vi "PID_2Chan_V4_Ramps.vi"() -> ()   [LabVIEW 2016]
uses:
  <vilib>/addons/control/pid/pid.llb/PID Advanced (DBL Array).vi
  <vilib>/addons/control/pid/pid.llb/PID Parameter Manager (DBL Array).vi
  <vilib>/addons/control/pid/pid.llb/PID Derivative Action Buffered (DBL Array).vi
  <vilib>/addons/control/pid/pid.llb/PID Get Advanced Error (DBL Array).vi
  <vilib>/addons/control/pid/pid.llb/PID Integral Action Buffered (DBL Array).vi
  <vilib>/addons/control/pid/pid.llb/PID Resize 1D Array.vi
  <vilib>/addons/control/pid/pid.llb/PID Get Advanced Error (DBL).vi
  <userlib>/Fluigent/Fluigent MFCS/FluigentMFCS_Full.llb/MFCS_EZ Detect.vi
  <userlib>/Fluigent/Fluigent MFCS/FluigentMFCS_Full.llb/MFCS_EZ Initialization.vi
  <userlib>/Fluigent/Fluigent MFCS/FluigentMFCS_Full.llb/MFCS_EZ Read All Channels Pressure.vi
  <userlib>/Fluigent/Fluigent MFCS/FluigentMFCS_Full.llb/MFCS_EZ Write Channel Pressure.vi
  <userlib>/Fluigent/Fluigent MFCS/FluigentMFCS_Full.llb/MFCS_EZ Close.vi
  <vilib>/addons/control/pid/NI_PID_pid.lvlib
  <vilib>/Analysis/NI_AALBase.lvlib
  <vilib>/Analysis/baseanly.llb/Mean (DBL).vi
panel:
  in  "setpoint profile":cluster{"time (s)":dbl, "setpoint":dbl}[](array[cluster]) {"setpoint" format="%.2f"; "time (s)" format="%.3f"}
  in  "Ramp?":bool
  in  "output cluster":T1
  out "Set Pressure":dbl[](array[numeric])=[400.0, 400.0]
  in  "linearity":dbl[](array[numeric])=[0.10000000000000003, 0.6000000000000001] format="%.2f"
  out "Flow 1 plot 2":cluster{"[0]":dbl, "[1]":dbl}(graph)={"[0]"=400.0, "[1]"=636.4874575000703}
  out "Flow Rates":dbl[](array[numeric])=[1099.9989421021717, 636.4874575000703]
  in  "FTot PID gains":cluster{"P":dbl, "I":dbl, "D":dbl}={"P"=0.01, "I"=0.0, "D"=0.0} {"D" format="%.6f"; "I" format="%.3f"; "P" format="%.5f"}
  in  "Ftot Setpoint":dbl=400.0
  in  "Vals to display":dbl=1235.0
  out "Flow 1 plot":cluster{"[0]":dbl, "[1]":dbl}(graph)={"[0]"=1099.9989421021717, "[1]"=300.0}
  out "Ferr":T2(graph)={"output[0]"=-2.2986299232843663, "output[1]"=-0.9866301071552578, "output[2]"=0.0}
  out "Pressures":dbl[](array[numeric])=[404.58697509765625, 396.3816223144531]
  in  "F1 PID gains":cluster{"P":dbl, "I":dbl, "D":dbl}={"P"=0.001, "I"=0.0, "D"=0.001} {"D" format="%.6f"; "I" format="%.3f"; "P" format="%.5f"}
  in  "reset Averging":bool
  in  "Set current Pressure\n to manual pressure":bool
  out "Pressures":T3(graph)={"[0]"=404.58697509765625, "[1]"=396.3816223144531, "[2]"=400.0, "[3]"=400.0}
  in  "stop":bool=TRUE
  in  "Control Valves":enum16{"1", "2", "3", "4", "5", "6", "7", "8"}[](array[ring])=[enum."7", enum."8"]
  in  "Pressure Channels":i16[](array[numeric])=[2, 3]
  in  "Manual Pressure Set":dbl[](array[numeric])=[400.0, 400.0] format="%_7g"
  in  "PID On":bool
  in  "reinitialize? (F)":bool
  in  "F1 Setpoint":dbl=300.0
  in  "Add Ctrl?":bool
  in  "Boards":enum16{"A", "B", "C"}[](array[ring])=[enum."A", enum."A"]
  in  "Valves":enum16{"1", "2", "3", "4", "5", "6", "7", "8"}[](array[ring])=[enum."5", enum."1"]
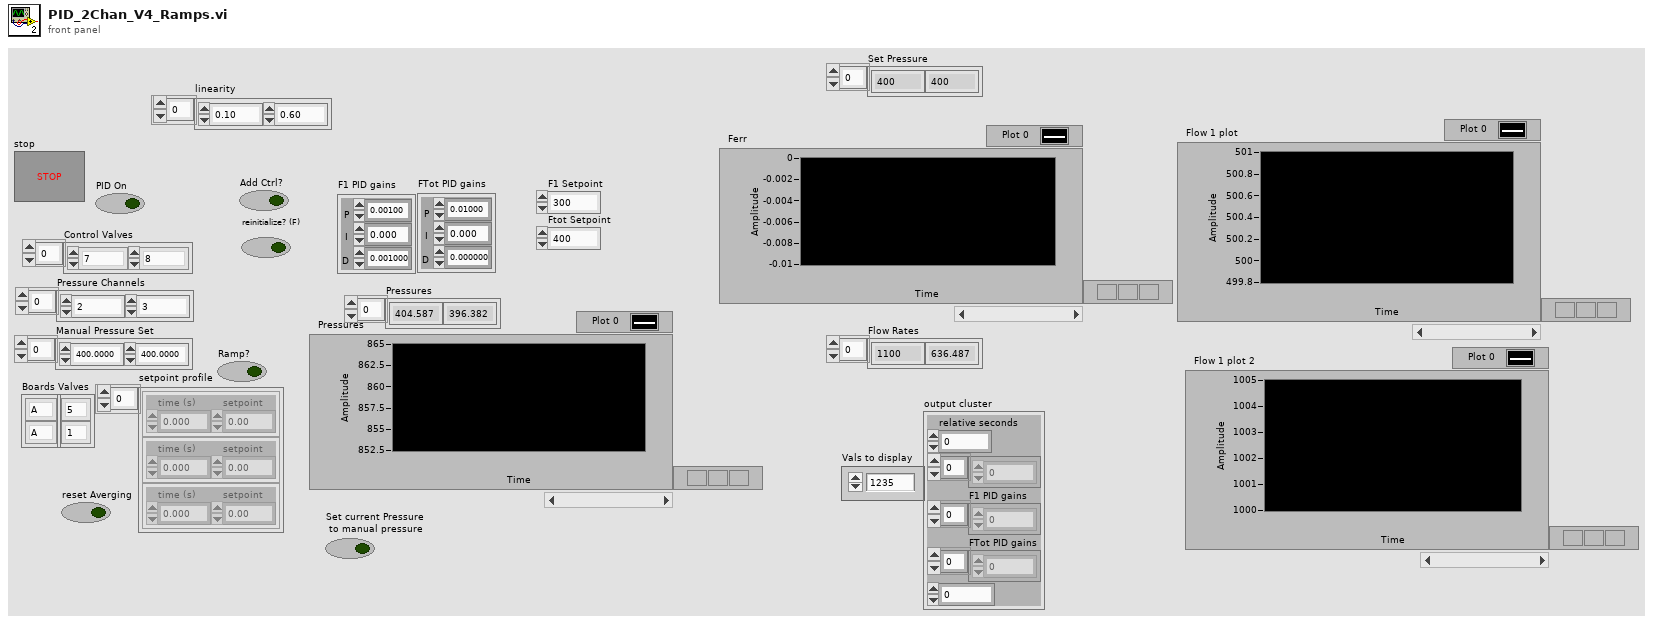
[diagram p1: front panel]
types:
  T1 = cluster{"relative seconds":dbl, "Pressures":dbl[], "F1 PID gains":dbl[], "FTot PID gains":dbl[], "PID On?":i16}
  T2 = cluster{"output[0]":dbl, "output[1]":dbl, "output[2]":dbl}
  T3 = cluster{"[0]":dbl, "[1]":dbl, "[2]":dbl, "[3]":dbl}
  T4 = cluster{"setpoint high":dbl, "setpoint low":dbl}[]
  T5 = typedef "_EZmfcsSN.ctl" = u16
  T6 = typedef "_EZmfcsRefNum.ctl" = refnum<k1>
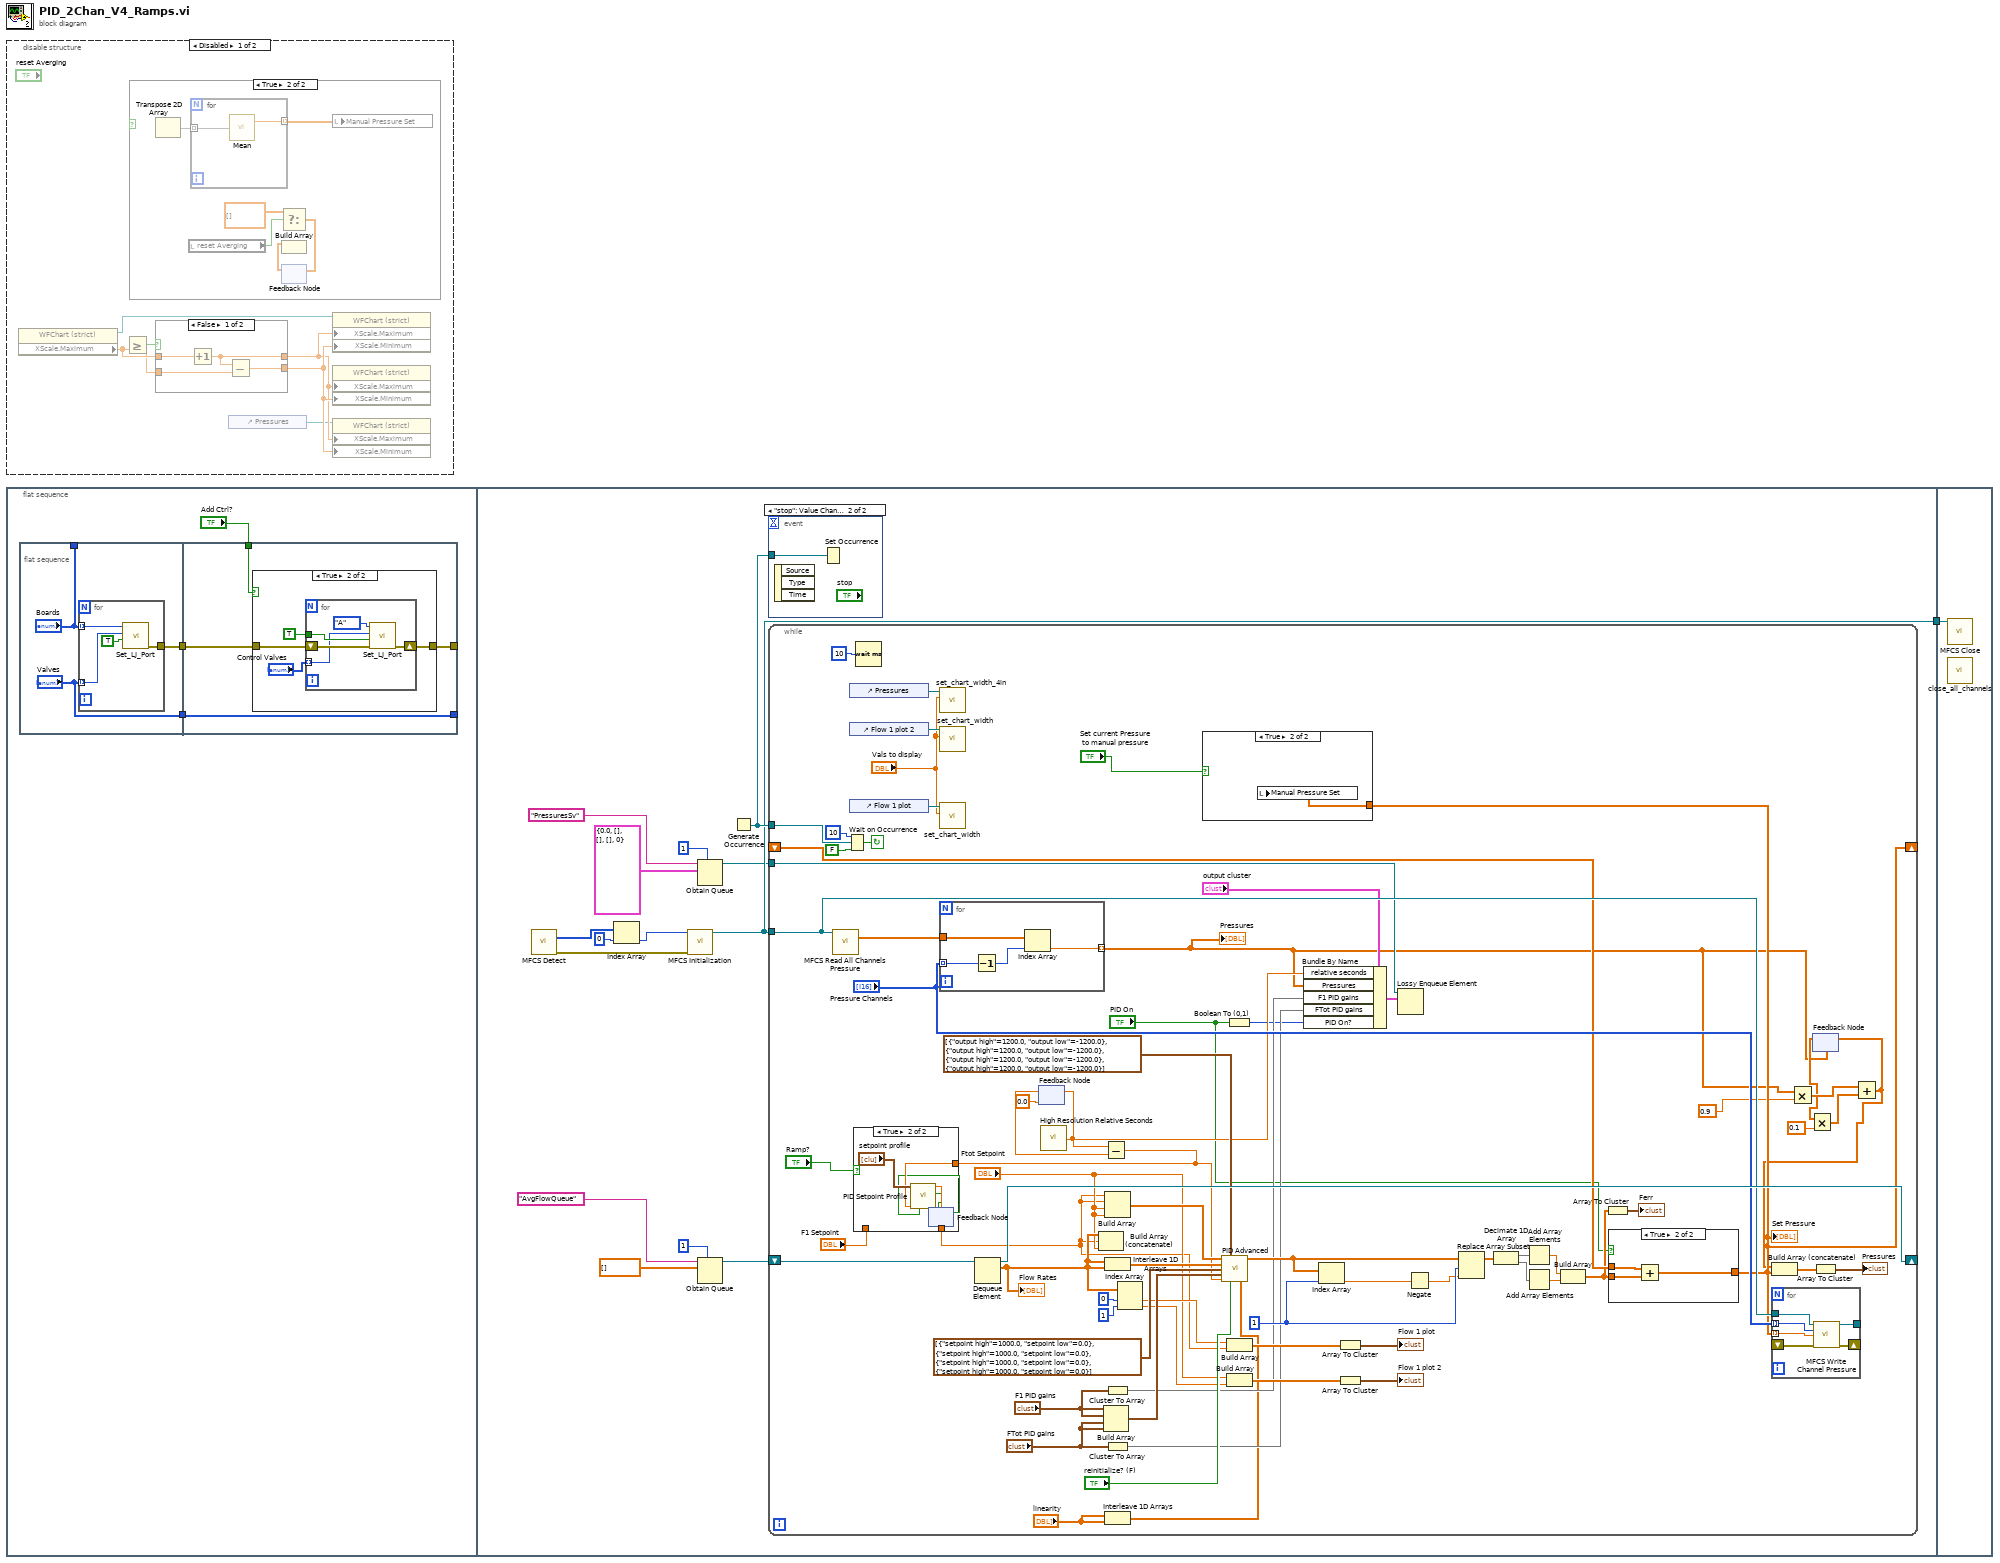
[diagram p0: block diagram]
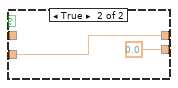
[diagram p2: hidden frame]
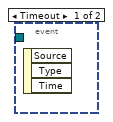
[diagram p6: hidden frame]
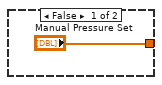
[diagram p9: hidden frame]
diagram:
  n1 = disable-structure shown="Disabled" {
    frame Disabled {
      n2 = property on="Property Node" class="WFChart (strict)"() -> (reference=w5:refnum<vi>, reference out=w6:refnum<vi>, "XScale.Maximum"=w4:dbl)  [unwired: 1 in, 1 out]
      n3 = Greater Or Equal?(y=w4) -> (x=w2:dbl, x >= y?=w3:bool)
      n4 = case shown="True" w11 {
        frame False {
        }
        frame True {
          n5 = Transpose 2D Array() -> (transposed array=w21:dbl[][])  [unwired: 1 in]
          n6 = local read "reset Averging"() -> (w22:bool)
          n7 = for {
            tunnel: w21 -> [w25] mode=indexing
            tunnel: [w24] -> w18 mode=indexing
            n8 = call-poly <vilib>:"Mean.vi"("X"=w25) -> ("mean"=w24:dbl)  [unwired: 1 out]
          }
          n9 = Select(t=dbl[][] [] ("appended array"), s=w22) -> (s? t:f=w19:dbl[][])  [unwired: 1 in]
          n10 = feedback-in #1(w19) -> ()
          n11 = feedback #1() -> (w23:dbl[][])  [unwired: 1 in]
          n12 = Build Array(w23) -> ()  [unwired: 1 in, 1 out]
          n13 = local write "Manual Pressure Set"(w18) -> ()
        }
      }
      n14 = case shown="False" w3 {
        tunnel: w2 -> [w13 w17]
        tunnel: w4 -> [w15 _]
        tunnel: [w12 w17] -> w9
        tunnel: [w14 0.0] -> w10
        frame False {
          n15 = Increment(x=w15) -> (x+1=w12:dbl)
          n16 = Subtract(x=w12, y=w13) -> (x-y=w14:dbl)
        }
        frame True {
        }
      }
      n17 = control-ref of="Pressures"() -> (w7:refnum<vi>)
      n18 = property on="Property Node" class="WFChart (strict)"(reference=w6, "XScale.Maximum"=w9, "XScale.Minimum"=w10) -> ()  [unwired: 1 in, 2 out]
      n19 = property on="Property Node" class="WFChart (strict)"("XScale.Maximum"=w9, "XScale.Minimum"=w10) -> (reference=w8:refnum<vi>)  [unwired: 1 in, 2 out]
      n20 = property on="Property Node" class="WFChart (strict)"(reference=w7, "XScale.Maximum"=w9, "XScale.Minimum"=w10) -> ()  [unwired: 1 in, 2 out]
    }
    frame Enabled {
    }
  }
  n21 = flat-sequence {
    tunnel: [w54] -> w1
    tunnel: w1 -> [w157]
    frame #0 {
      n22 = flat-sequence {
        tunnel: ["Boards"] -> _
        tunnel: [w31] -> w28
        tunnel: ["Valves"] -> w27
        tunnel: [w39] -> _
        tunnel: [w37] -> _
        tunnel: w28 -> [w38]
        tunnel: w27 -> [w39]
        tunnel: "Add Ctrl?" -> [w36]
        frame #0 {
          n23 = for {
            tunnel: "Valves" -> [w35] mode=indexing
            tunnel: "Boards" -> [w34] mode=indexing
            tunnel: [w32] -> w31
            n24 = call "Set_LJ_Port.vi"("State"=TRUE, "Channel"=w35, "Flowboard"=w34) -> ("error out"=w32:errorcluster)  [unwired: 8 in]
          }
        }
        frame #1 {
          n25 = case shown="True" w36 {
            tunnel: w38 -> [w40 w44]
            tunnel: [w40 w43] -> w37
            frame False {
            }
            frame True {
              n26 = for {
                tunnel: TRUE ("State") -> [w47]
                shift-right: [w48] -> w43
                shift-left: w44 -> [w49]
                tunnel: "Control Valves" -> [w46] mode=indexing
                n27 = call "Set_LJ_Port.vi"("error in"=w49, "State"=w47, "Channel"=w46, "Flowboard"=enum16{"A", "B", "C"}."A") -> ("error out"=w48:errorcluster)  [unwired: 7 in]
              }
            }
          }
        }
      }
    }
    frame #1 {
      n28 = call-poly <userlib>:"MFCS Detect.vi"() -> ("[SN MFCS_EZ]"=w63:T5[], "error out"=w61:errorcluster)  [unwired: 14 in]
      n29 = Index Array(array=w63, index=0) -> (element=w62:T5)
      n30 = call-poly <userlib>:"MFCS Initialization.vi"("SN MFCS_EZ"=w62, "error in (no error)"=w61) -> ("MFCS_EZ"=w54:T6)  [unwired: 11 in, 2 out]
      n31 = Obtain Queue(max queue size (-1, unlimited)=1, name (unnamed)="PressuresSv", element data type=T1 {"relative seconds"=0.0, "Pressures"=[], "F1 PID gains"=[], "FTot PID gains"=[], "PID On?"=0} ("output cluster")) -> (queue out=w52:refnum<queue>)  [unwired: 2 in, 2 out]
      n32 = Obtain Queue(max queue size (-1, unlimited)=1, name (unnamed)="AvgFlowQueue", element data type=dbl[] [] ("appended array")) -> (queue out=w57:refnum<queue>)  [unwired: 2 in, 2 out]
      n33 = Generate Occurrence() -> (w56:refnum<k4>)
      n34 = event shown="[1] \"stop\": Value Change" {
        selector: _ -> [_ _]
        dyn-events: _ -> [_ _]
        timeout: _ -> [_ _]
        tunnel: w56 -> [_ w64]
        event Timeout {
          n35 = event-data() -> ()  [unwired: 1 in, 3 out]
        }
        event "stop": Value Change {
          n36 = event-data() -> ()  [unwired: 1 in, 3 out]
          n37 = Set Occurrence(w64) -> ()
        }
      }
      n38 = while {
        shift-right: [w134] -> _
        shift-left: w57 -> [w135]
        tunnel: w56 -> [w121]
        tunnel: w54 -> [w110]
        shift-right: [w73] -> _
        shift-left: _ -> [w105]
        tunnel: w52 -> [w96]
        stop <- w120 continue-if-true
        w128 = 1 ("index")
        n39 = call-poly <userlib>:"MFCS Read All Channels Pressure.vi"("MFCS_EZ"=w110) -> ("All Channels Pressure"=w108:dbl[])  [unwired: 12 in, 2 out]
        n40 = Wait on Occurrence(1:FALSE ("ignore previous (T)"), 2:w121, 3:10 ("ms timeout (-1)")) -> (0:w120:bool)
        n41 = control-ref of="Pressures"() -> (w107:refnum<vi>)
        n42 = control-ref of="Flow 1 plot 2"() -> (w90:refnum<vi>)
        n43 = control-ref of="Flow 1 plot"() -> (w89:refnum<vi>)
        n44 = Wait (ms)(milliseconds to wait=u32 10) -> ()  [unwired: 1 out]
        n45 = call "set_chart_width_4in.vi"("Values to Display"="Vals to display", "Ref In"=w107) -> ()  [unwired: 10 in]
        n46 = call "set_chart_width.vi"("Values to Display"="Vals to display", "Ref In"=w90) -> ()  [unwired: 10 in]
        n47 = call "set_chart_width.vi"("Values to Display"="Vals to display", "Ref In"=w89) -> ()  [unwired: 10 in]
        n48 = for {
          tunnel: "Pressure Channels" -> [w145] mode=indexing
          tunnel: w108 -> [w146]
          tunnel: [w143] -> w65 mode=indexing
          n49 = Decrement(x=w145) -> (x-1=w144:i16)
          n50 = Index Array(array=w146, index=w144) -> (element=w143:dbl)
        }
        "Pressures" <- w65
        n51 = Dequeue Element(queue=w135) -> (queue out=w134:refnum<queue>, element=w101:dbl[])  [unwired: 2 in, 2 out]
        "Flow Rates" <- w101
        n52 = feedback #2(0.0 ("relative seconds")) -> (w130:dbl)
        n53 = call <vilib>:"High Resolution Relative Seconds.vi"() -> ("relative seconds"=w95:dbl)
        n54 = feedback-in #2(w95) -> ()
        n55 = Subtract(x=w95, y=w130) -> (x-y=w77:dbl)
        n56 = case shown="True" "Ramp?" {
          tunnel: w77 -> [_ w141]
          tunnel: [w137 w140] -> w76
          tunnel: "F1 Setpoint" -> [w137 _]
          frame False {
          }
          frame True {
            n57 = feedback #3() -> (w138:bool)  [unwired: 1 in]
            n58 = call <vilib>:"PID Setpoint Profile.vi"("reinitialize? (F)"=w138, "dt (s)"=w141, "setpoint profile"="setpoint profile") -> ("profile complete?"=w139:bool, "setpoint"=w140:dbl)  [unwired: 3 in, 2 out]
            n59 = feedback-in #3(w139) -> ()
          }
        }
        n60 = Build Array (concatenate)(w101, w76, "Ftot Setpoint") -> ()  [unwired: 1 out]
        n61 = Build Array("F1 PID gains", "F1 PID gains", "FTot PID gains", "FTot PID gains") -> (w124:cluster{"P":dbl, "I":dbl, "D":dbl}[])
        n62 = Build Array(w76, w76, "Ftot Setpoint", "Ftot Setpoint") -> (w118:dbl[])
        n63 = Interleave 1D Arrays(w101, w101) -> (w112:dbl[])
        n64 = Cluster To Array(cluster="F1 PID gains") -> (array=w94:dbl[])
        n65 = Cluster To Array(cluster="FTot PID gains") -> (array=w93:dbl[])
        n66 = Interleave 1D Arrays("linearity", "linearity") -> (w81:dbl[])
        n67 = Index Array(array=w101, index #1=0 ("index"), index #2=1 ("index")) -> (element #1=w87:dbl, element #2=w85:dbl)
        n68 = call-poly <vilib>:"PID Advanced.vi"("setpoint"=w118, "output range"=cluster{"output high":dbl, "output low":dbl}[] [{"output high"=1200.0, "output low"=-1200.0}, {"output high"=1200.0, "output low"=-1200.0}, {"output high"=1200.0, "output low"=-1200.0}, {"output high"=1200.0, "output low"=-1200.0}], "process variable"=w112, "setpoint range"=T4 [{"setpoint high"=1000.0, "setpoint low"=0.0}, {"setpoint high"=1000.0, "setpoint low"=0.0}, {"setpoint high"=1000.0, "setpoint low"=0.0}, {"setpoint high"=1000.0, "setpoint low"=0.0}], "PID gains"=w124, "dt (s)"=w77, "reinitialize? (F)"="reinitialize? (F)", "linearity"=w81) -> ("output"=w125:dbl[])  [unwired: 6 in, 1 out]
        n69 = Boolean To (0,1)(Boolean="PID On") -> (0, 1=w91:i16)
        n70 = Build Array(w87, w76) -> (w100:dbl[])
        n71 = Build Array("Ftot Setpoint", w85) -> (w98:dbl[])
        n72 = Bundle By Name(cluster="output cluster", "relative seconds"=w95, "Pressures"=w65, "F1 PID gains"=w94, "FTot PID gains"=w93, "PID On?"=w91) -> (w79:T1)
        n73 = Index Array(array=w125, index=w128) -> (element=w127:dbl)
        n74 = Array To Cluster(array=w100) -> (cluster=→"Flow 1 plot":cluster{"[0]":dbl, "[1]":dbl})
        n75 = Array To Cluster(array=w98) -> (cluster=→"Flow 1 plot 2":cluster{"[0]":dbl, "[1]":dbl})
        n76 = Lossy Enqueue Element(queue=w96, element=w79) -> ()  [unwired: 1 in, 4 out]
        n77 = Negate(x=w127) -> (-x=w126:dbl)
        n78 = Replace Array Subset(array=w125, new element=w126, index=w128) -> (w117:dbl[])
        n79 = Decimate 1D Array(w117) -> (w116:dbl[], w115:dbl[])
        n80 = Add Array Elements(numeric array=w116) -> (sum=w114:dbl)
        n81 = Add Array Elements(numeric array=w115) -> (sum=w113:dbl)
        n82 = Build Array(w114, w113) -> (w104:dbl[])
        n83 = Array To Cluster(array=w104) -> (cluster=→"Ferr":cluster{"[0]":dbl, "[1]":dbl, "[2]":dbl})
        n84 = case shown="True" "PID On" {
          tunnel: w104 -> [_ w156]
          tunnel: w105 -> [_ w155]
          tunnel: ["Manual Pressure Set" w154] -> w73
          frame False {
          }
          frame True {
            n85 = Add(x=w155, y=w156) -> (x+y=w154:dbl[])
          }
        }
        "Set Pressure" <- w73
        n86 = case shown="True" "Set current Pressure\n to manual pressure" {
          tunnel: w73 -> [_ w136]
          frame False {
          }
          frame True {
            n87 = local write "Manual Pressure Set"(w136) -> ()
          }
        }
        n88 = for {
          shift-right: [w151] -> _
          shift-left: _ -> [w152]
          tunnel: [w150] -> _
          tunnel: "Pressure Channels" -> [w149] mode=indexing
          tunnel: w73 -> [w148] mode=indexing
          tunnel: w110 -> [w147]
          n89 = call-poly <userlib>:"MFCS Write Channel Pressure.vi"("MFCS_EZ"=w147, "Channel Number (default=1)"=w149, "Pressure (mBar)"=w148, "error in (no error)"=w152) -> ("MFCS_EZ out"=w150:T6, "error out"=w151:errorcluster)  [unwired: 10 in]
        }
        n90 = Multiply(x=w65, y=0.9) -> (x*y=w70:dbl[])
        n91 = feedback #4(w65) -> (w68:dbl[])
        n92 = Multiply(x=w68, y=0.1) -> (x*y=w67:dbl[])
        n93 = Add(x=w70, y=w67) -> (x+y=w66:dbl[])
        n94 = Build Array (concatenate)(w66, w73) -> (w72:dbl[])
        n95 = feedback-in #4(w66) -> ()
        n96 = Array To Cluster(array=w72) -> (cluster=→"Pressures":T3)
      }
    }
    frame #2 {
      n97 = call-poly <userlib>:"MFCS Close.vi"("MFCS_EZ"=w157) -> ()  [unwired: 14 in, 1 out]
      n98 = call "close_all_channels.vi"() -> ()  [unwired: 12 in]
    }
  }
